vi "Set UI Vals.vi"(10 "UI Vals":map{string, cluster{"New?":bool, variant}}(c390), 11 "Series UI Actor in":refnum<class "Series UI Actor.lvclass">) -> (3 "Series UI Actor out":refnum<class "Series UI Actor.lvclass">)   [LabVIEW 2024, in "Series UI Actor.lvlib" / "Series UI Actor.lvclass"]
uses:
  Series UI Actor.lvclass
  Series UI Actor.lvclass/Series UI Actor.ctl
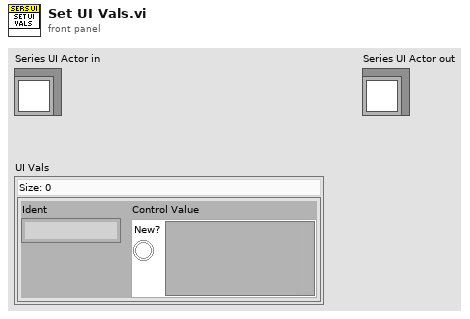
[diagram p1: front panel]
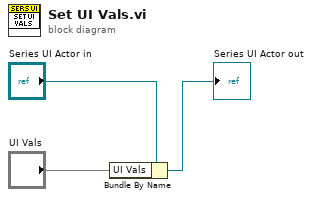
[diagram p0: block diagram]
diagram:
  n1 = Bundle By Name(cluster="Series UI Actor in", "UI Vals"="UI Vals") -> (→"Series UI Actor out":refnum<class "Series UI Actor.lvclass">)
